vi "FA_ApplyRTEXE.vi"(8 "Error In":errorcluster) -> (0 "Error Out":errorcluster)   [LabVIEW 2014, in "FA_ApplyRTEXE.lvlib"]
uses:
  FA_ApplyRTEXE.lvlib
  FA_NativeTypes API/source/VI Source/FA_Config.ctl
  FA_LocalStore API/source/VI Source/FA_LSSpecialTypes.ctl
  <vilib>/nisyscfg/Close (System).vi
  FA_LocalStore API/source/VI Source/FA_LocalStore.lvlib
  FA_NativeTypes API/source/VI Source/FA_NativeTypes.lvlib
  <vilib>/nisyscfg/nisyscfg.lvlib
panel:
  out "ConfigData":T1
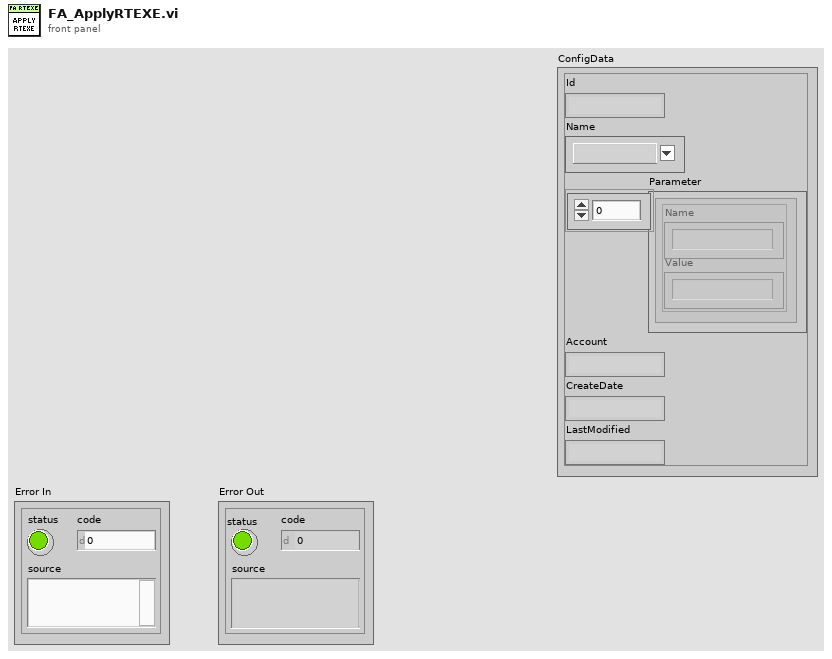
[diagram p1: front panel]
types:
  T1 = typedef "FA_NativeTypes.lvlib/FA_Config.ctl" = cluster{"Id":string, "Name":T2, "Parameter":cluster{"Name":string, "Value":string}[], "Account":string, "CreateDate":string, "LastModified":string}
  T2 = typedef "FA_LocalStore.lvlib/FA_LSSpecialTypes.ctl" = string
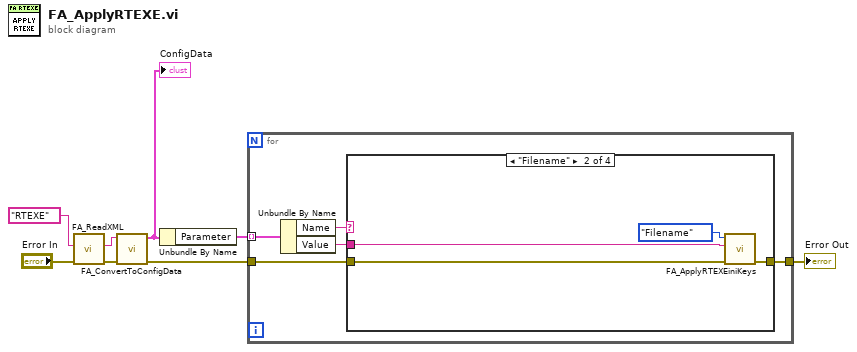
[diagram p0: block diagram]
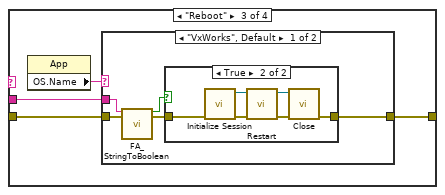
[diagram p3: hidden frame]
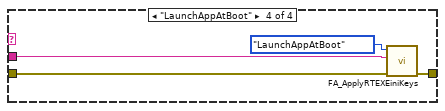
[diagram p6: hidden frame]
diagram:
  n1 = call "FA_ReadXML.vi"("Error In"="Error In", "Special Type"=T2 "RTEXE") -> ("Error Out"=w5:errorcluster, "XML String"=w6:string)  [unwired: 6 in]
  n2 = call "FA_ConvertToConfigData.vi"("Error In"=w5, "XML String"=w6) -> ("Error Out"=w2:errorcluster, "ConfigData"=w4:T1)  [unwired: 8 in]
  "ConfigData" <- w4
  n3 = Unbundle By Name(w4) -> ("Parameter"=w3:cluster{"Name":string, "Value":string}[])
  n4 = for {
    tunnel: w3 -> [w13] mode=indexing
    tunnel: w2 -> [w10]
    tunnel: [w9] -> w1
    n5 = Unbundle By Name(w13) -> ("Name"=w12:string, "Value"=w11:string)
    n6 = case shown="\"Filename\"" w12 {
      tunnel: w11 -> [_ w16 w20 w39]
      tunnel: w10 -> [w14 w18 w21 w37]
      tunnel: [w14 w17 w19 w36] -> w9
      frame "False", Default {
      }
      frame "Filename" {
        n7 = call "FA_ApplyRTEXEiniKeys.vi"("Error In"=w18, "Value In"=w16, "INI Key Type"=enum16{"Filename", "LaunchAppAtBoot"}."Filename") -> ("Error Out"=w17:errorcluster)  [unwired: 8 in]
      }
      frame "Reboot" {
        n8 = property class="App"() -> ("OS.Name"=w22:string)  [unwired: 2 in, 2 out]
        n9 = case shown="\"VxWorks\", Default" w22 {
          tunnel: [w27 w35] -> w19
          tunnel: w21 -> [w26 w35]
          tunnel: w20 -> [w25 _]
          frame "VxWorks", Default {
            n10 = call "FA_StringToBoolean.vi"("Input String"=w25, "Error In"=w26) -> ("Boolean"=w23:bool, "Error Out"=w24:errorcluster)  [unwired: 16 in]
            n11 = case shown="True" w23 {
              tunnel: [w28 w30] -> w27
              tunnel: w24 -> [w28 w29]
              frame False {
              }
              frame True {
                n12 = call <vilib>:"Initialize Session.vi"("error in (no error)"=w29) -> ("error out"=w32:errorcluster, "Session out"=w34:refnum<k21>)  [unwired: 9 in]
                n13 = call <vilib>:"Restart.vi"("error in (no error)"=w32, "Session in"=w34) -> ("error out"=w31:errorcluster, "Session out"=w33:refnum<k21>)  [unwired: 7 in, 1 out]
                n14 = call-poly <vilib>:"Close.vi"("error in (no error)"=w31, "Session in"=w33) -> ("error out"=w30:errorcluster)  [unwired: 9 in]
              }
            }
          }
          frame "Windows NT" {
            # "Don't call reboot\nfunctions when on\nthe dev machine"
          }
        }
      }
      frame "LaunchAppAtBoot" {
        n15 = call "FA_ApplyRTEXEiniKeys.vi"("Error In"=w37, "Value In"=w39, "INI Key Type"=enum16{"Filename", "LaunchAppAtBoot"}."LaunchAppAtBoot") -> ("Error Out"=w36:errorcluster)  [unwired: 8 in]
      }
    }
  }
  "Error Out" <- w1
